vi "Read Digital In.vi"(8 "error in (no error)":errorcluster, 10 "Pin":u8 max=7 step=1, 11 "VISA resource name":refnum<visa-resource-name>) -> (0 "error out":errorcluster, 2 "state (F: Off)":bool, 3 "VISA resource name out":refnum<visa-resource-name>)   [LabVIEW 2022 SP3, in "usbtmc_scpi_labtool.lvlib"]
uses:
  usbtmc_scpi_labtool.lvlib
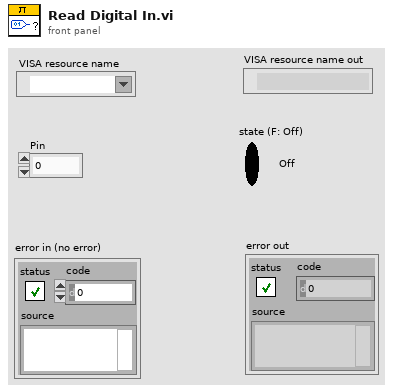
[diagram p1: front panel]
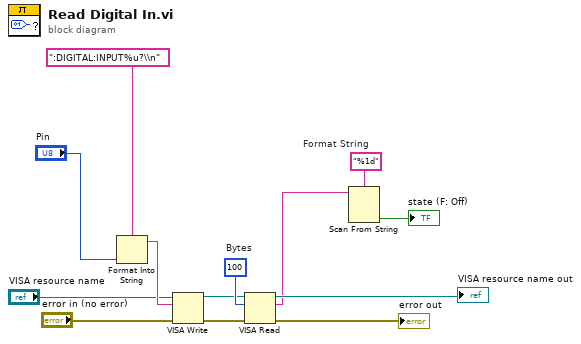
[diagram p0: block diagram]
diagram:
  w7 = "%1d"  # Format String
  w8 = u32 100  # Bytes
  n1 = Format Into String(format string=":DIGITAL:INPUT%u?\\n", "Pin") -> (resulting string=w12:string)  [unwired: 2 in, 1 out]
  n2 = VISA Write(VISA resource name="VISA resource name", write buffer=w12, error in (no error)="error in (no error)") -> (VISA resource name out=w4:refnum<visa-resource-name>, error out=w5:errorcluster)  [unwired: 1 out]
  n3 = VISA Read(VISA resource name=w4, byte count=w8, error in (no error)=w5) -> (VISA resource name out=→"VISA resource name out":refnum<visa-resource-name>, read buffer=w1:string, error out=→"error out":errorcluster)  [unwired: 1 out]
  n4 = Scan From String(format string=w7, input string=w1) -> (output 1=→"state (F: Off)":bool)  [unwired: 3 in, 3 out]
